vi "flash_firmware.vi"(6 "timeout (25000ms)":i32=25000, 7 "SW 4.1 and above?":bool, 8 "error in (no error)":errorcluster, 9 "SIV bin path":path, 10 "firmware path":path, 11 "daemon reference in":refnum<k5>) -> (0 "error out":errorcluster, 2 "response":string, 3 "daemon reference out":refnum<k5>, 5 "command out":string="random")   [LabVIEW 2017]
doc: "<b>Command: </b>\"template\"\n\n<b>Description: </b> This command does something.\n\n<b>Parameters: </b> None\n____________________________________________\nDIPC 692 Daemon API 10.0.0.1\nSam Tee - Dyson Technology Ltd\nCopyright (c) 2024, Dyson Technology Ltd"
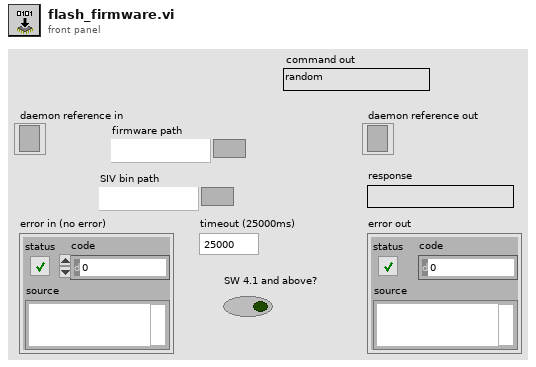
[diagram p1: front panel]
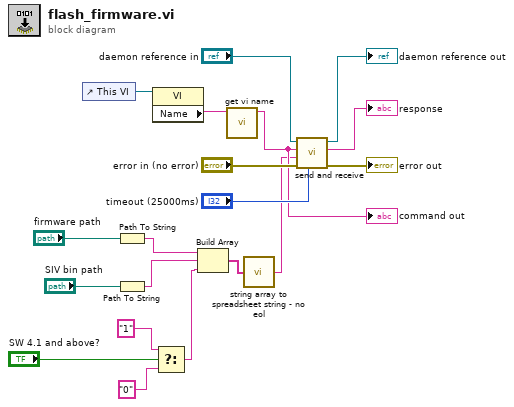
[diagram p0: block diagram]
diagram:
  n1 = control-ref of="This VI"() -> (w13:refnum<vi>)
  n2 = Path To String(path="firmware path") -> (string=w8:string)
  n3 = Path To String(path="SIV bin path") -> (string=w7:string)
  n4 = property class="VI"(reference=w13) -> ("Name"=w12:string)  [unwired: 1 in, 2 out]
  n5 = Select(t="1", s="SW 4.1 and above?", f="0") -> (s? t:f=w1:string)
  n6 = Build Array(w8, w7, w1) -> (w6:string[])
  n7 = call "get vi name.vi"("library.lvlib:name.vi"=w12) -> ("vi name"=w11:string)  [unwired: 10 in]
  "command out" <- w11
  n8 = call "string array to spreadsheet string - no eol.vi"("string array"=w6) -> ("spreadsheet string - no eol"=w5:string)
  n9 = call "send and receive.vi"("timeout (25000ms)"="timeout (25000ms)", "error in (no error)"="error in (no error)", "data"=w5, "command"=w11, "daemon reference in"="daemon reference in") -> ("error out"=→"error out":errorcluster, "response"=→"response":string, "daemon reference out"=→"daemon reference out":refnum<k5>)  [unwired: 4 in]
